vi "Bodies_Force2Torque.vi"(8 "error in (no error)":errorcluster, 10 "Force":T1, 11 "Bodies.lvclass":refnum<class "Bodies.lvclass">) -> (0 "error out":errorcluster, 1 "FpInGCS":dbl[](array[numeric]) format="%#.6f", 2 "Torque Vector":dbl[](array[numeric]), 3 "Bodies.lvclass 2":refnum<class "Bodies.lvclass">)   [LabVIEW 2015, in "Bodies.lvclass"]
uses:
  Bodies.lvclass
  Force.ctl
  PointOnBody.ctl
  <vilib>/Analysis/BLAS.llb/LV_Transpose.ctl
  <vilib>/Analysis/Matrix/Numeric/Conversions/Array To Matrix - RA2.vi
  <vilib>/Analysis/BLAS.llb/dgemv - General Matrix-Vector Product (DBL).vi
  <vilib>/Analysis/Matrix/NI_Matrix.lvlib
  <vilib>/Analysis/NI_AALBLAS.lvlib
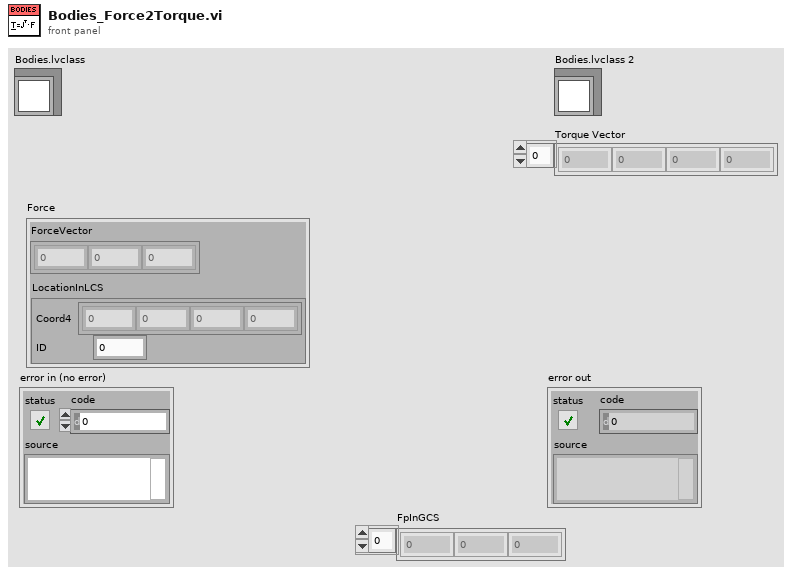
[diagram p1: front panel]
types:
  T1 = typedef "Bodies.lvclass/Force.ctl" = cluster{"LocationInLCS":T2, "ForceVector":dbl[]}
  T2 = typedef "Bodies.lvclass/PointOnBody.ctl" = cluster{"Coord4":dbl[], "ID":i32}
  T3 = typedef "NI_AALBLAS.lvlib/LV_Transpose.ctl" = i32
  T4 = typedef "NI_Matrix.lvlib/RealMatrix.ctl" = dbl[][]
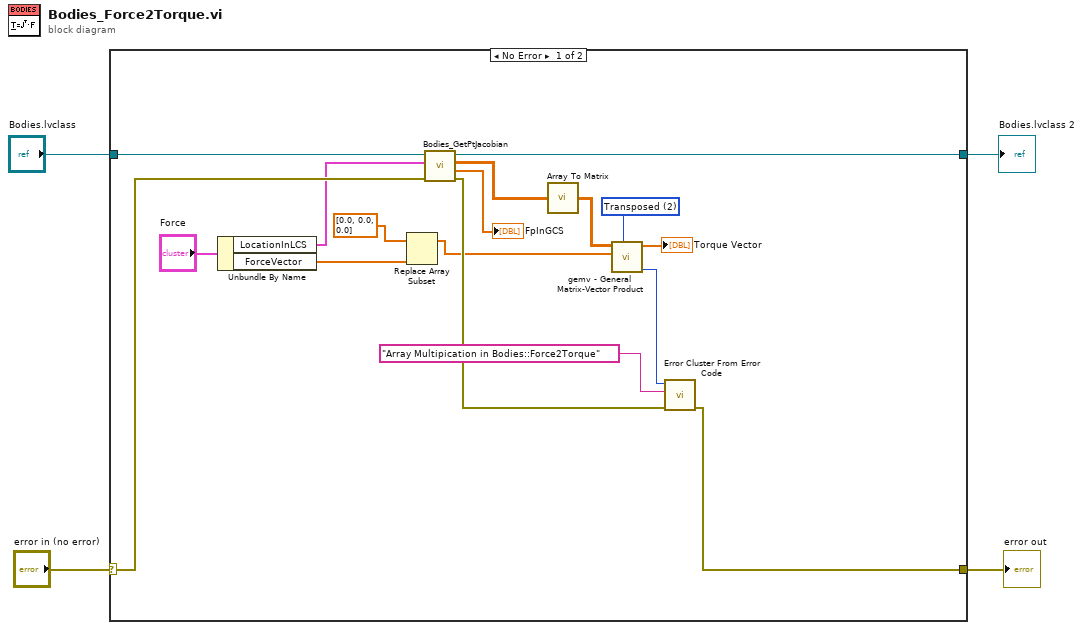
[diagram p0: block diagram]
diagram:
  n1 = case shown="No Error" "error in (no error)" {
    selector: "error in (no error)" -> [w20 w23]
    tunnel: "Bodies.lvclass" -> [w21 w22]
    tunnel: [w12 w23] -> w3
    tunnel: [w15 w22] -> w1
    frame No Error {
      w5 = T3 2 items=["Direct", "Conjugated & Transposed", "Transposed"] ("operation A")
      n2 = Unbundle By Name("Force") -> ("LocationInLCS"=w18:T2, "ForceVector"=w8:dbl[])
      n3 = Replace Array Subset(array=dbl[] [0.0, 0.0, 0.0], new element=w8) -> (w7:dbl[])  [unwired: 1 in]
      n4 = call "Bodies_GetPtJacobian.vi"("error in (no error)"=w20, "Point"=w18, "Bodies.lvclass"=w21) -> ("error out"=w13:errorcluster, "PointInGCS"=→"FpInGCS":dbl[], "Jacobian"=w6:dbl[][], "Bodies.lvclass 2"=w15:refnum<class "Bodies.lvclass">)  [unwired: 5 in]
      n5 = call-poly <vilib>:"Array To Matrix.vi"("Real 2D Array"=w6) -> ("Real Matrix"=w17:T4)
      n6 = call-poly <vilib>:"gemv - General Matrix-Vector Product.vi"("operation A"=w5, "x"=w7, "A"=w17) -> ("error"=w14:i32, "dgemv"=→"Torque Vector":dbl[])  [unwired: 7 in]
      n7 = call <vilib>:"Error Cluster From Error Code.vi"("error in (no error)"=w13, "error message (\"\")"="Array Multipication in Bodies::Force2Torque" ("error source (\" \")"), "error code (0)"=w14) -> ("error out"=w12:errorcluster)  [unwired: 6 in]
    }
    frame Error {
    }
  }
  "error out" <- w3
  "Bodies.lvclass 2" <- w1
